vi "New Input poller Event.vi"(8 "error in (no error)":errorcluster) -> (0 "error out":errorcluster, 2 "result_event":refnum<user-event>, 3 "input_poller_event out":refnum<class "input_poller_event.lvclass">)   [LabVIEW 2015, in "input_poller_event.lvclass"]
uses:
  input_poller_event.lvclass
  Result/result.lvclass
  input_poller_event.lvclass/input_poller_event.ctl
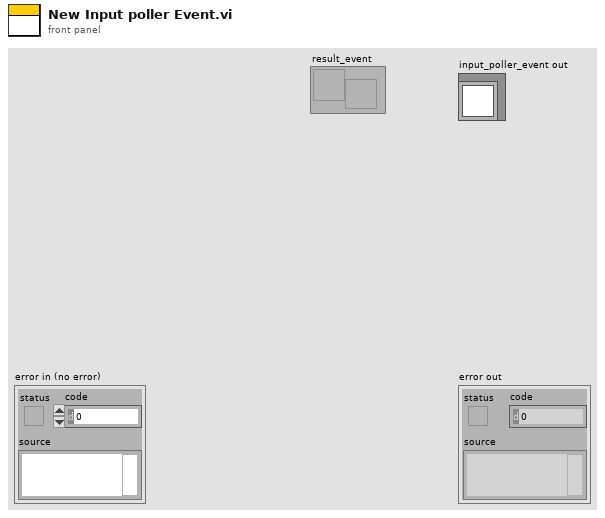
[diagram p1: front panel]
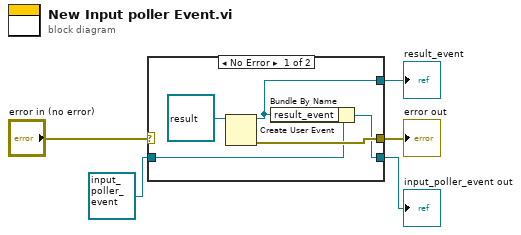
[diagram p0: block diagram]
diagram:
  n1 = case shown="No Error" "error in (no error)" {
    selector: "error in (no error)" -> [_ w12]
    tunnel: [w10 w12] -> w4
    tunnel: [w7 w11] -> w2
    tunnel: refnum<class "input_poller_event.lvclass"> refnum ("input_poller_event in") -> [w8 w11]
    tunnel: [w6 _] -> w1
    frame No Error {
      n2 = Create User Event(user event datatype=refnum<class "result.lvclass"> refnum ("result.lvclass")) -> (user event=w6:refnum<user-event>, error out=w10:errorcluster)  [unwired: 1 in]
      n3 = Bundle By Name(cluster=w8, "result_event"=w6) -> (w7:refnum<class "input_poller_event.lvclass">)
    }
    frame Error {
    }
  }
  "error out" <- w4
  "input_poller_event out" <- w2
  "result_event" <- w1
